vi "pack_raw.vi"(3 "error in":errorcluster, 4 "data":u8[](array[numeric]), 5 "p":u64) -> (0 "error out":errorcluster, 2 "p out":u64)   [LabVIEW 2019, in "msgpack.lvlib"]
doc: "Packs a raw data stream (stored as a U8 array) into the msgpack buffer.\n\nUse the pack_item VI to pack a raw data string."
uses:
  msgpack.lvlib
  msgpackalt.dll
panel:
  # "msgpack"
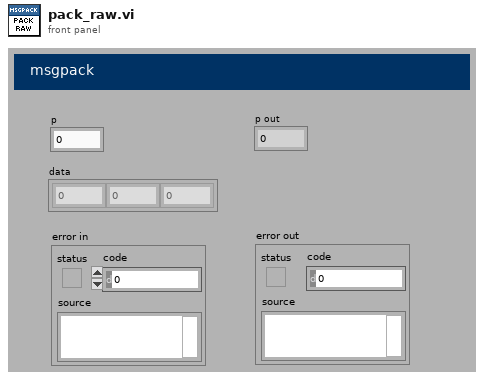
[diagram p1: front panel]
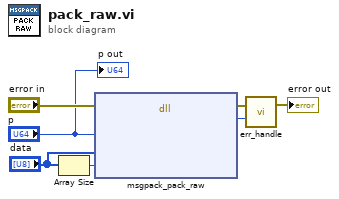
[diagram p0: block diagram]
diagram:
  n1 = Array Size(array="data") -> (size(s)=w5:i32)
  n2 = dll-call lib="C:/Users/Patrick/Documents/GitHub/Instrument-Framework/lvsrc/SMOs/JSON-RPC-2019/lv-venv/lv.lib/vi.lib/addons/msgpack/msgpackalt.dll" fn="msgpack_pack_raw"(error in="error in", "p"="p", "x"="data", "len"=w5) -> (error out=w2:errorcluster, "return type"=w3:i32)  [unwired: 5 in, 1 out]
  n3 = call "err_handle.vi"("retval"=w3, "error in"=w2) -> ("error out"=→"error out":errorcluster)  [unwired: 1 in]
  "p out" <- "p"
